vi "PH_HamamatsuCamera.search Cam.vi"(2 "Wanted Cam":string, 4 "Cam Error in":errorcluster) -> (13 "Cam found":bool, 15 "Available Cams":string[](array[string]), 16 "Handle":i32, 17 "Camera Details":T1, 18 "Cam Error out":errorcluster)   [LabVIEW 2014, in "PH_HamamatsuCamera.lvlib"]
uses:
  PH_HamamatsuCamera.lvlib
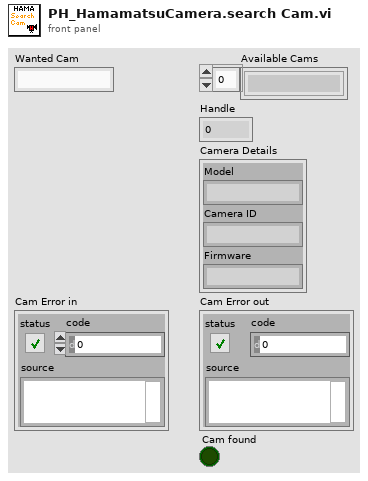
[diagram p1: front panel]
types:
  T1 = cluster{"Model":string, "Camera ID":string, "Firmware":string}
  T2 = cluster{"Model":string, "Camera ID":string, "Firmware":string}[]
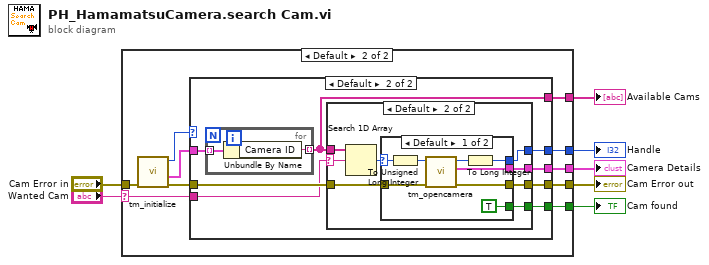
[diagram p0: block diagram]
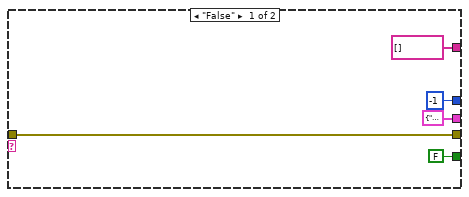
[diagram p2: hidden frame]
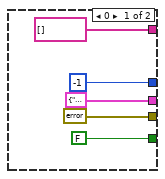
[diagram p3: hidden frame]
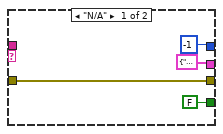
[diagram p4: hidden frame]
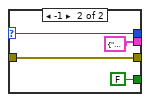
[diagram p5: hidden frame]
diagram:
  n1 = case shown="Default" "Wanted Cam" {
    selector: "Wanted Cam" -> [_ w13]
    tunnel: [FALSE w22] -> w7
    tunnel: [string[] [] w21] -> w6
    tunnel: [T1 {"Model"="", "Camera ID"="", "Firmware"=""} ("Camera Details") w20] -> w5
    tunnel: "Cam Error in" -> [w9 w19]
    tunnel: [w9 w18] -> w3
    tunnel: [-1 ("index of element") w15] -> w2
    frame "False" {
    }
    frame Default {
      n2 = call <userlib>:"tm_initialize.vi"("error in (no error)"=w19) -> ("error out"=w16:errorcluster, "Camera Details Array"=w14:T2, "Number Of Cameras"=w17:u32)  [unwired: 7 in, 1 out]
      n3 = case shown="Default" w17 {
        tunnel: w14 -> [_ w29]
        tunnel: [-1 ("index of element") w35] -> w15
        tunnel: w16 -> [_ w34]
        tunnel: [T1 {"Model"="", "Camera ID"="", "Firmware"=""} ("Camera Details") w33] -> w20
        tunnel: [errorcluster {"status"=FALSE, "code"=0, "source"=""} ("error out") w32] -> w18
        tunnel: [FALSE w31] -> w22
        tunnel: w13 -> [_ w30]
        tunnel: [string[] [] w28] -> w21
        frame 0 {
        }
        frame Default {
          n4 = for {
            tunnel: w29 -> [w37] mode=indexing
            tunnel: [w36] -> w28 mode=indexing
            n5 = Unbundle By Name(w37) -> ("Camera ID"=w36:string)
          }
          n6 = case shown="Default" w30 {
            selector: w30 -> [_ w47]
            tunnel: [-1 ("index of element") w48] -> w35
            tunnel: w34 -> [w40 w46]
            tunnel: [T1 {"Model"="", "Camera ID"="", "Firmware"=""} ("Camera Details") w44] -> w33
            tunnel: [w40 w45] -> w32
            tunnel: [FALSE w43] -> w31
            tunnel: w28 -> [_ w42]
            frame "N/A" {
            }
            frame Default {
              n7 = Search 1D Array(1D array=w42, element=w47) -> (index of element=w49:i32)  [unwired: 1 in]
              n8 = case shown="Default" w49 {
                selector: w49 -> [w57 w61]
                tunnel: [w51 w61] -> w48
                tunnel: w46 -> [w55 w60]
                tunnel: [w53 w60] -> w45
                tunnel: [w52 T1 {"Model"="", "Camera ID"="", "Firmware"=""} ("Camera Details")] -> w44
                tunnel: [TRUE FALSE] -> w43
                frame Default {
                  n9 = To Unsigned Long Integer(number=w57) -> (unsigned 32bit integer=w56:u32)
                  n10 = call <userlib>:"tm_opencamera.vi"("error in (no error)"=w55, "Camera Index"=w56) -> ("error out"=w53:errorcluster, "Camera Details"=w52:T1, "Handle out"=w54:u32)  [unwired: 7 in]
                  n11 = To Long Integer(number=w54) -> (32bit integer=w51:i32)
                }
                frame -1 {
                }
              }
            }
          }
        }
      }
    }
  }
  "Cam found" <- w7
  "Available Cams" <- w6
  "Camera Details" <- w5
  "Cam Error out" <- w3
  "Handle" <- w2
